vi "Init Writes Buffer.vi"(8 "error in":errorcluster, 11 "BufferWrites1SamDBL in":refnum<class "BufferWrites1SamDBL.lvclass">) -> (0 "error out":errorcluster, 3 "BufferWrites1SamDBL out":refnum<class "BufferWrites1SamDBL.lvclass">)   [LabVIEW 2023, in "BufferWrites1SamDBL.lvclass"]
uses:
  BufferWrites1SamDBL.lvclass
  BufferWrites1SamDBL.lvclass/BufferWrites1SamDBL.ctl
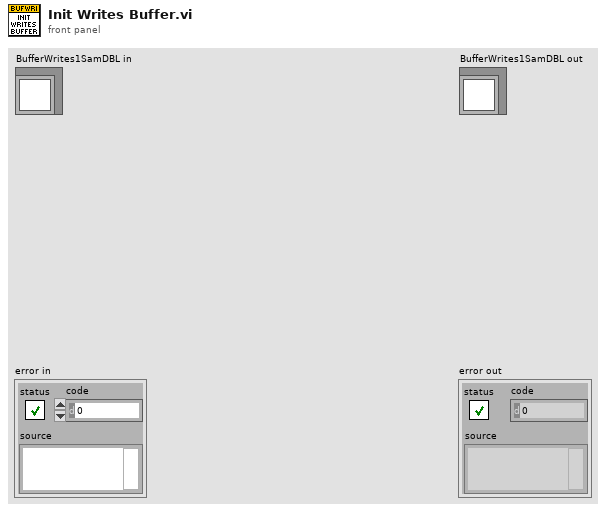
[diagram p1: front panel]
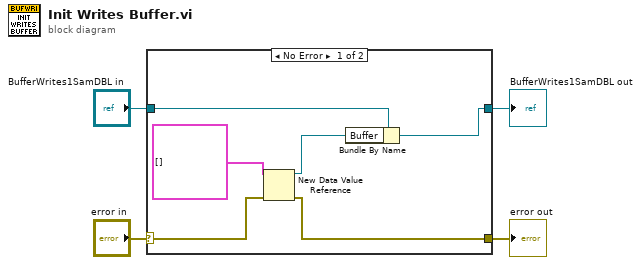
[diagram p0: block diagram]
diagram:
  n1 = case shown="No Error" "error in" {
    selector: "error in" -> [w7 w12]
    tunnel: [w6 w12] -> w3
    tunnel: [w9 w11] -> w1
    tunnel: "BufferWrites1SamDBL in" -> [w10 w11]
    frame No Error {
      n2 = New Data Value Reference(data value=cluster{"Ident":string, "Value":dbl}[] [], error in=w7) -> (data value reference=w5:refnum<data-value>, error out=w6:errorcluster)
      n3 = Bundle By Name(cluster=w10, "Buffer"=w5) -> (w9:refnum<class "BufferWrites1SamDBL.lvclass">)
    }
    frame Error {
    }
  }
  "error out" <- w3
  "BufferWrites1SamDBL out" <- w1
